vi "Configure UL-DL Pattern.vi"(4 "No Of UL Symbols (4)":i32=4, 5 "No Of UL Slots (4)":i32=4, 6 "No Of DL Symbols (4)":i32=4, 7 "No Of DL Slots (3)":i32=3, 8 "error in (no error)":errorcluster, 9 "SCS (30 kHz)":i32(ring)=1 items=["15 kHz", "30 kHz", "60 kHz"], 10 "Instance (1)":T1=1, 11 "VISA resource name":refnum<visa-resource-name>) -> (0 "error out":errorcluster, 3 "VISA resource name out":refnum<visa-resource-name>)   [LabVIEW 2020, in "Rohde&Schwarz CMWXP NR FR1 Measurement.lvlib"]
doc: "Configures the UL-DL pattern for the <SCSpacing>.\n\nAttribute:\nRSCMWXPNRFR1M_ATTR_UL_DL_PATTERN\n\nRemote-control command:\nCONFigure:NRSub:MEAS<i>:ULDL:PATTern"
uses:
  <instrlib>/Rohde&Schwarz CMWXP NR FR1 Measurement/Rohde&Schwarz CMWXP NR FR1 Measurement.lvlib
  <instrlib>/Rohde&Schwarz CMWXP NR FR1 Measurement/Private/_Instance.ctl
  <instrlib>/Rohde&Schwarz CMWXP NR FR1 Measurement/Private/rsidr_core.llb/rsidr_core.lvlib
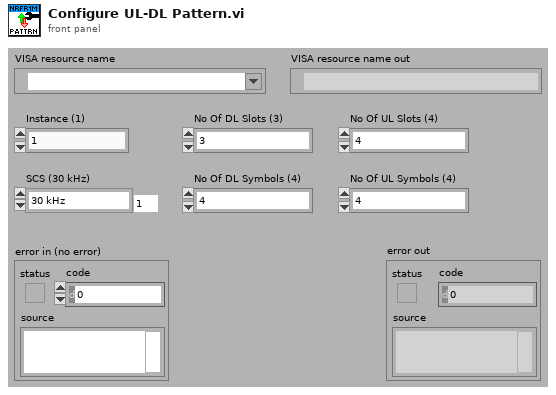
[diagram p1: front panel]
types:
  T1 = typedef "Rohde&Schwarz CMWXP NR FR1 Measurement.lvlib/_Instance.ctl" = i32
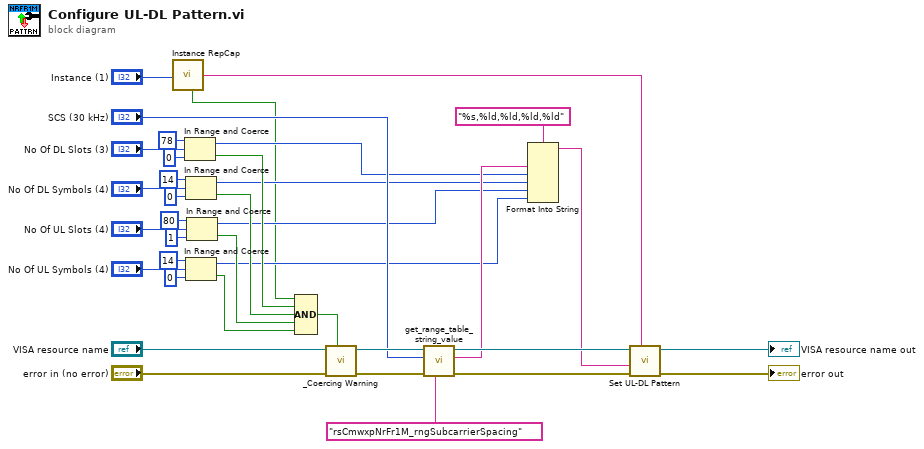
[diagram p0: block diagram]
diagram:
  n1 = call <instrlib>:"Instance RepCap.vi"("Instance In"="Instance (1)") -> ("In Range?"=w1:bool, "RepCap Identifier Out"=w2:string)  [unwired: 1 in]
  n2 = In Range and Coerce(upper limit=78, x="No Of DL Slots (3)", lower limit=0) -> (coerced(x)=w7:i32, In Range?=w21:bool)
  n3 = In Range and Coerce(upper limit=14, x="No Of DL Symbols (4)", lower limit=0) -> (coerced(x)=w6:i32, In Range?=w22:bool)
  n4 = In Range and Coerce(upper limit=14, x="No Of UL Symbols (4)", lower limit=0) -> (coerced(x)=w4:i32, In Range?=w24:bool)
  n5 = In Range and Coerce(upper limit=80, x="No Of UL Slots (4)", lower limit=1) -> (coerced(x)=w5:i32, In Range?=w23:bool)
  n6 = Compound Arithmetic op=AND(w1, w21, w22, w23, w24) -> (w20:bool)
  n7 = call <instrlib>:"_Coercing Warning.vi"("In Range?"=w20, "error in (no error)"="error in (no error)", "VISA resource name"="VISA resource name") -> ("error out"=w17:errorcluster, "VISA resource name out"=w16:refnum<visa-resource-name>)  [unwired: 7 in]
  n8 = call <instrlib>:"get_range_table_string_value.vi"("Range Table ID in"="rsCmwxpNrFr1M_rngSubcarrierSpacing", "error in"=w17, "I32 input"="SCS (30 kHz)", "VISA resource name"=w16) -> ("error out"=w15:errorcluster, "String Value out"=w8:string, "VISA resource name out"=w12:refnum<visa-resource-name>)  [unwired: 5 in]
  n9 = Format Into String(format string="%s,%ld,%ld,%ld,%ld", w8, w7, w6, w5, w4) -> (resulting string=w3:string)  [unwired: 2 in, 1 out]
  n10 = call "Set UL-DL Pattern"("Repeated Capabilities"=w2, "error in (no error)"=w15, "UL-DL Pattern ()"=w3, "instrument handle"=w12) -> ("error out"=→"error out":errorcluster, "instrument handle out"=→"VISA resource name out":refnum<visa-resource-name>)  [unwired: 6 in]
